vi "Read Boolean.vi"(8 "error in (no error)":errorcluster, 11 "dependencyData in":refnum<class "dependencyData.lvclass">) -> (0 "error out":errorcluster, 2 "Boolean":bool, 3 "dependencyData out":refnum<class "dependencyData.lvclass">)   [LabVIEW 2020, in "eos.lvlib" / "dependencyData.lvclass"]
uses:
  dependencyData.lvclass
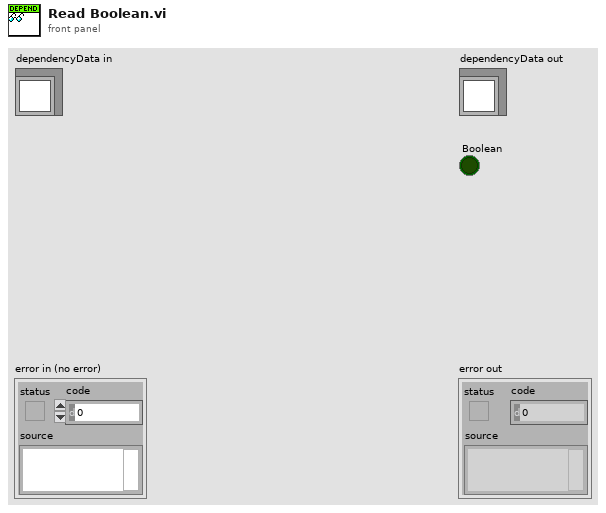
[diagram p1: front panel]
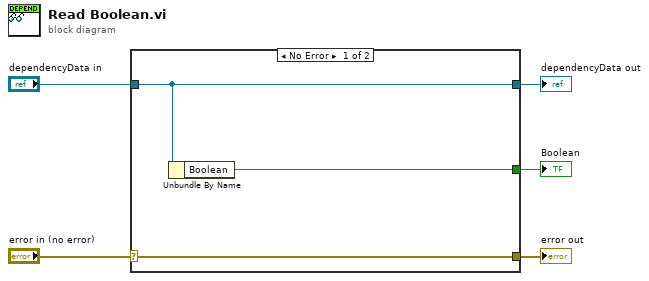
[diagram p0: block diagram]
diagram:
  n1 = case shown="No Error" "error in (no error)" {
    selector: "error in (no error)" -> [w8 w9]
    tunnel: [w8 w9] -> w4
    tunnel: [w7 w10] -> w2
    tunnel: "dependencyData in" -> [w7 w10]
    tunnel: [w6 _] -> w1
    frame No Error {
      n2 = Unbundle By Name(w7) -> ("Boolean"=w6:bool)
    }
    frame Error {
    }
  }
  "error out" <- w4
  "dependencyData out" <- w2
  "Boolean" <- w1
